vi "Close.vi"(8 "error in (no error)":errorcluster, 11 "StepperController in":refnum<class "StepperController.lvclass">) -> (0 "error out":errorcluster, 3 "StepperController out":refnum<class "StepperController.lvclass">)   [LabVIEW 2013, in "StepperController.lvclass"]
uses:
  StepperController.lvclass
  StepperController.lvclass/StepperController.ctl
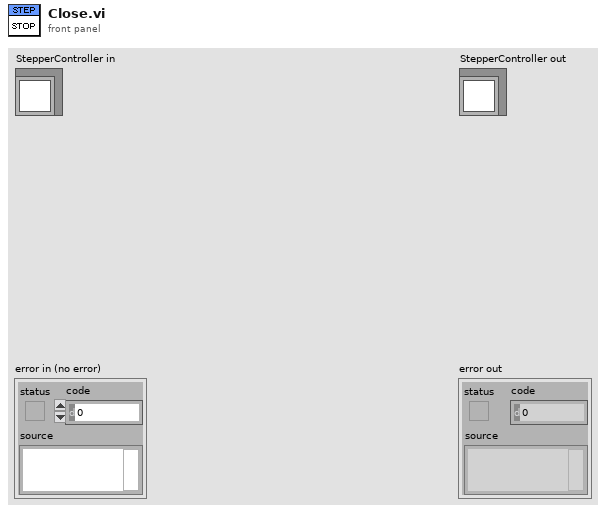
[diagram p1: front panel]
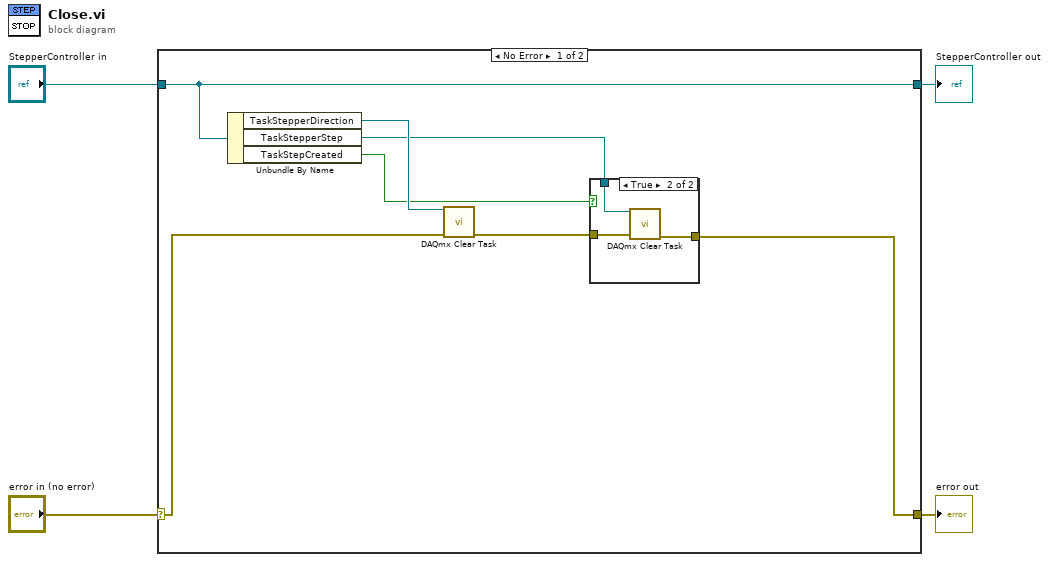
[diagram p0: block diagram]
diagram:
  n1 = case shown="No Error" "error in (no error)" {
    selector: "error in (no error)" -> [w7 w16]
    tunnel: [w6 w16] -> w3
    tunnel: [w11 w17] -> w1
    tunnel: "StepperController in" -> [w11 w17]
    frame No Error {
      n2 = Unbundle By Name(w11) -> ("TaskStepperDirection"=w10:refnum<k21>, "TaskStepperStep"=w9:refnum<k21>, "TaskStepCreated"=w5:bool)
      n3 = call <vilib>:"DAQmx Clear Task.vi"("task in"=w10, "error in"=w7) -> ("error out"=w8:errorcluster)  [unwired: 13 in]
      n4 = case shown="True" w5 {
        tunnel: w9 -> [_ w15]
        tunnel: w8 -> [w12 w14]
        tunnel: [w12 w13] -> w6
        frame False {
        }
        frame True {
          n5 = call <vilib>:"DAQmx Clear Task.vi"("task in"=w15, "error in"=w14) -> ("error out"=w13:errorcluster)  [unwired: 13 in]
        }
      }
    }
    frame Error {
    }
  }
  "error out" <- w3
  "StepperController out" <- w1
